vi "getCount.vi"(8 "error in (no error)":errorcluster, 11 "IEnumerationType in":refnum<class "IEnumerationType.lvclass">) -> (0 "error out":errorcluster, 2 "Count out":i32, 3 "IEnumerationType out":refnum<class "IEnumerationType.lvclass">)   [LabVIEW 2022 SP3, in "openDAQ.lvlib" / "daqCoreTypes.lvlib" / "IEnumerationType.lvclass"]
uses:
  <instrlib>/openDAQ/Public/Classes/daqCoreTypes/IEnumerationType/IEnumerationType.lvclass
  <instrlib>/openDAQ/Public/Classes/daqCoreTypes/IEnumerationType/IEnumerationType.lvclass/IEnumerationType.ctl
  <instrlib>/openDAQ/Binaries/Windows/x86/copendaq32.dll
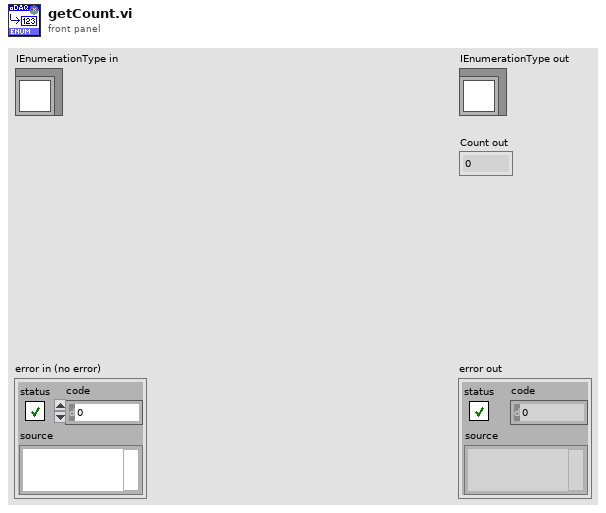
[diagram p1: front panel]
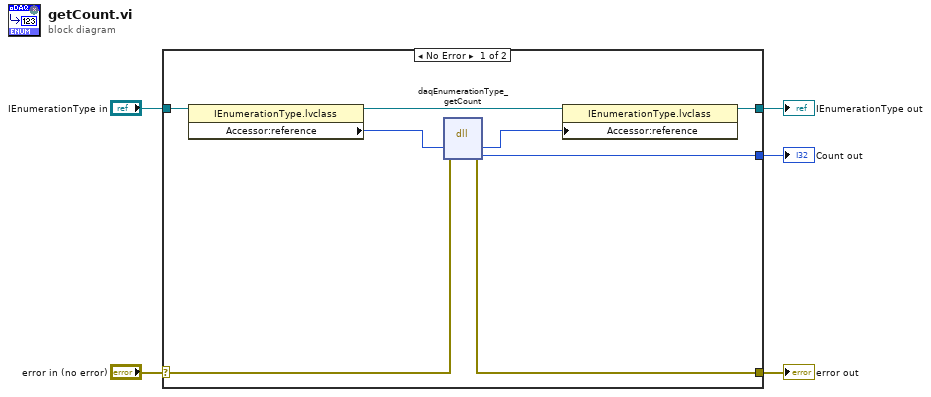
[diagram p0: block diagram]
diagram:
  n1 = case shown="No Error" "error in (no error)" {
    selector: "error in (no error)" -> [w12 w15]
    tunnel: [w11 w15] -> w4
    tunnel: [w9 w14] -> w2
    tunnel: "IEnumerationType in" -> [w13 w14]
    tunnel: [w6 _] -> w1
    frame No Error {
      n2 = property class="IEnumerationType.lvclass"(reference=w13) -> (reference out=w10:refnum<class "IEnumerationType.lvclass">, "Accessor:reference"=w8:i64)  [unwired: 1 in, 1 out]
      n3 = dll-call lib="C:/Program Files (x86)/National Instruments/LabVIEW 2022/instr.lib/openDAQ/Binaries/Windows/x86/copendaq*.*" fn="daqEnumerationType_getCount"(error in=w12, "enumerationType"=w8) -> (error out=w11:errorcluster, "enumerationType"=w7:i64, "count"=w6:i32)  [unwired: 4 in, 1 out]
      n4 = property class="IEnumerationType.lvclass"(reference=w10, "Accessor:reference"=w7) -> (reference out=w9:refnum<class "IEnumerationType.lvclass">)  [unwired: 1 in, 1 out]
    }
    frame Error {
    }
  }
  "error out" <- w4
  "IEnumerationType out" <- w2
  "Count out" <- w1
